vi "多参数测量数据存储.vi"(5 "数据类型":string(combo)="N", 6 "手动启动标记":bool, 7 "测量模式":T2(ring)=enum."水样测试", 8 "error in (no error)":errorcluster, 9 "database":string, 10 "table输入":string, 11 "data in":T1) -> (0 "error out":errorcluster)   [LabVIEW 2016, in "斯坦道多参数.lvlib"]
uses:
  <vilib>/Utility/sysdir.llb/System Directory Type.ctl
  <vilib>/Utility/error.llb/DialogType.ctl
  <vilib>/addons/database/Auxilliary.llb/DB Tools Transaction.ctl
  <vilib>/addons/database/Auxilliary.llb/DB Tools Isolation Level.ctl
  <vilib>/addons/database/Connection.llb/DB Tools Open Connec (String).vi
  <vilib>/addons/database/Connection.llb/Conn Execute.vi
  <vilib>/addons/database/Recordset.llb/Rec Destroy - Connection.vi
  <vilib>/addons/database/Connection.llb/Conn Transaction.vi
  <vilib>/addons/database/NI_Database_API.lvlib
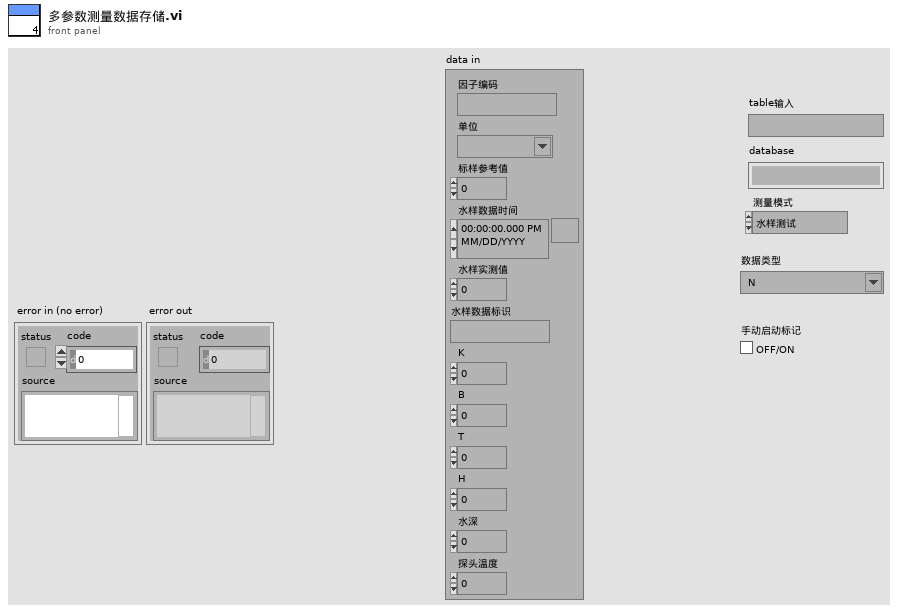
[diagram p1: front panel]
types:
  T1 = cluster{"因子编码":string, "单位":string, "标样参考值":sgl, "水样数据时间":timestamp, "水样实测值":sgl, "水样数据标识":string, "K":sgl, "B":sgl, "T":sgl, "H":sgl, "水深":sgl, "探头温度":sgl}
  T2 = enum16{"待机", "水样测试", "标样核查", "零点核查", "跨度核查", "空白测试", "平行样测试", "加标回收", "空白校准", "标样校准", "初始化（清洗）"}
  T3 = typedef "NI_Database_API.lvlib/DB Tools Transaction.ctl" = enum16{"begin", "commit", "rollback"}
  T4 = typedef "NI_Database_API.lvlib/DB Tools Isolation Level.ctl" = enum16{"chaos", "read uncommitted", "read committed", "repeatable read", "serializable"}
  T5 = typedef "DialogType.ctl" = u16
  T6 = typedef "System Directory Type.ctl" = i32
  T7 = cluster{"时间标识":timestamp, "测量模式":string, "数据类型":string, "监测值":sgl, "单位":string, "数据标识":string, "因子编码":string, "标样参考值":sgl, "K":sgl, "B":sgl, "温度":sgl, "湿度":sgl, "水深":sgl, "探头温度":sgl, "LastTime":timestamp}
  T8 = typedef "NI_Database_API.lvlib/Conn ObjectReference.ctl" = refnum<k1>
  T9 = typedef "NI_Database_API.lvlib/Rec ObjectReference.ctl" = refnum<k1>
  T10 = cluster{"时间标识":timestamp, "设备":string, "日志信息":string}
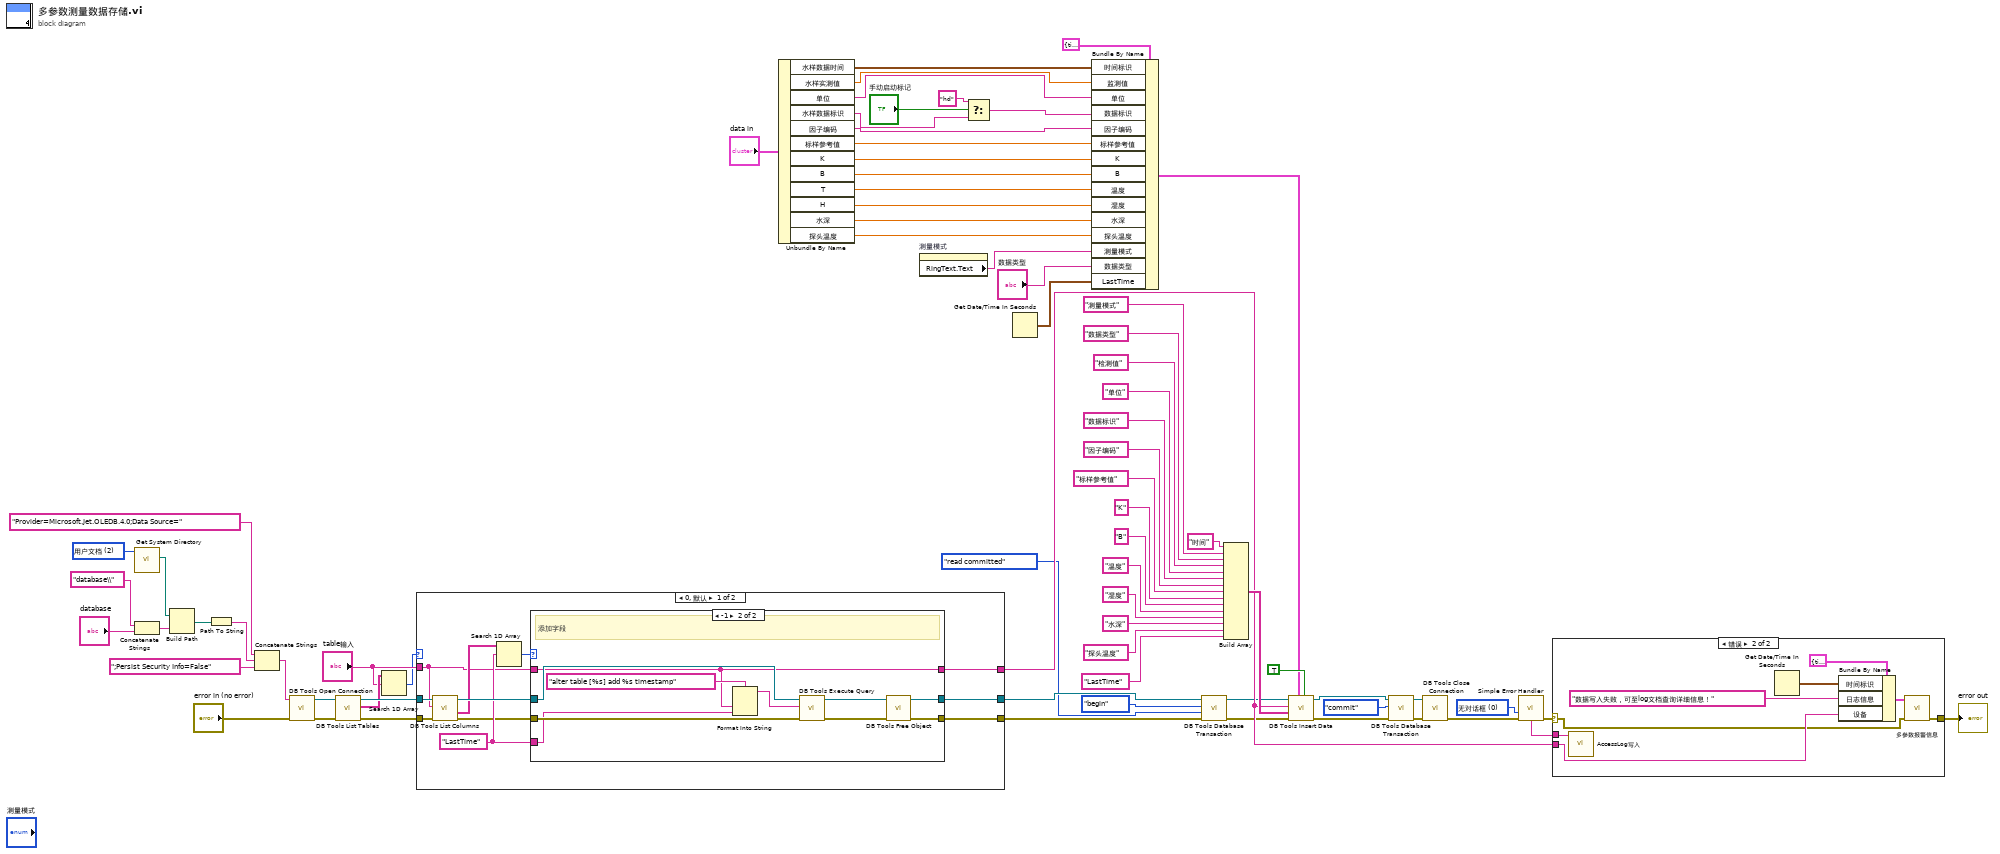
[diagram p0: block diagram]
diagram:
  w27 = T5 0 items=["无对话框", "确定信息", "继续或停止信息", "确定信息＋警告", "继续/停止+警告"] ("type of dialog (OK msg:1)")
  w47 = T6 2 items=["用户目录"=0, "用户桌面"=1, "用户文档"=2, "用户应用程序数据"=3, "用户设置"=4, "用户临时目录"=5, "公共文档"=6, "公共应用程序数据"=7, "公共设置"=8, "公共缓存"=13, "系统核心库"=9, "系统安装库"=10, "应用程序文件"=11, "启动盘根目录"=12] ("system directory type")
  n1 = call <vilib>:"Get System Directory.vi"("system directory type"=w47) -> ("system directory"=w45:path)  [unwired: 10 in]
  n2 = Concatenate Strings("database\\" ("condition"), "database") -> (w39:string)
  n3 = Build Path(base path=w45, name or relative path=w39) -> (appended path=w44:path)
  n4 = Path To String(path=w44) -> (string=w43:string)
  n5 = Concatenate Strings("Provider=Microsoft.Jet.OLEDB.4.0;Data Source=" ("condition"), w43, ";Persist Security Info=False" ("condition")) -> (w41:string)
  n6 = call-poly <vilib>:"DB Tools Open Connection.vi"("error in (no error)"="error in (no error)", "connection information"=w41) -> ("error out"=w18:errorcluster, "connection reference"=w29:T8)  [unwired: 6 in]
  n7 = call <vilib>:"DB Tools List Tables.vi"("error in (no error)"=w18, "connection reference"=w29) -> ("error out"=w17:errorcluster, "tables"=w16:string[], "connection reference out"=w19:T8)  [unwired: 3 in]
  n8 = Search 1D Array(1D array=w16, element="table输入") -> (index of element=w14:i32)  [unwired: 1 in]
  n9 = case shown="0, 默认" w14 {
    tunnel: [w79 w100] -> w28
    tunnel: [w78 w98] -> w10
    tunnel: [w77 w99] -> w22
    tunnel: w19 -> [w76 w100]
    tunnel: w17 -> [w75 w98]
    tunnel: "table输入" -> [w74 w99]
    frame 0, Default {
      w83 = "LastTime" ("元素")
      n10 = call <vilib>:"DB Tools List Columns.vi"("error in (no error)"=w75, "table"=w74, "connection reference"=w76) -> ("error out"=w81:errorcluster, "columns"=w82:string[], "connection reference out"=w84:T8)  [unwired: 1 in, 1 out]
      n11 = Search 1D Array(1D array=w82, element=w83) -> (index of element=w80:i32)  [unwired: 1 in]
      n12 = case shown="-1" w80 {
        tunnel: w84 -> [w87 w95]
        tunnel: w81 -> [w86 w94]
        tunnel: w83 -> [_ w92]
        tunnel: [w87 w90] -> w79
        tunnel: [w86 w89] -> w78
        tunnel: w74 -> [w85 w88]
        tunnel: [w85 w88] -> w77
        frame 0, Default {
        }
        frame -1 {
          # "添加字段"
          n13 = Format Into String(format string="alter table [%s] add %s timestamp", w88, w92) -> (resulting string=w91:string)  [unwired: 2 in, 1 out]
          n14 = call-poly <vilib>:"DB Tools Execute Query.vi"("error in (no error)"=w94, "SQL query"=w91, "connection reference"=w95) -> ("error out"=w96:errorcluster, "recordset reference"=w97:T9)  [unwired: 5 in]
          n15 = call-poly <vilib>:"DB Tools Free Object.vi"("error in (no error)"=w96, "recordset reference"=w97) -> ("error out"=w89:errorcluster, "connection reference"=w90:T8)  [unwired: 8 in]
        }
      }
    }
    frame -1 {
    }
  }
  n16 = Unbundle By Name("data in") -> ("水样数据时间"=w64:timestamp, "水样实测值"=w63:sgl, "单位"=w56:string, "水样数据标识"=w1:string, "因子编码"=w55:string, "标样参考值"=w57:sgl, "K"=w58:sgl, "B"=w62:sgl, "T"=w61:sgl, "H"=w60:sgl, "水深"=w35:sgl, "探头温度"=w32:sgl)
  n17 = property on="测量模式" class="Enum (严格)"() -> ("RingText.Text"=w54:string)  [unwired: 2 in, 2 out]
  n18 = Select(t="hd", s="手动启动标记", f=w1) -> (s? t:f=w3:string)
  n19 = Get Date/Time In Seconds() -> (seconds since 1Jan1904=w21:timestamp)
  n20 = Bundle By Name(cluster=T7 {"时间标识"=timestamp(0 s since 1904-01-01), "测量模式"="", "数据类型"="", "监测值"=0.0, "单位"="", "数据标识"="", "因子编码"="", "标样参考值"=0.0, "K"=0.0, "B"=0.0, "温度"=0.0, "湿度"=0.0, "水深"=0.0, "探头温度"=0.0, "LastTime"=timestamp(0 s since 1904-01-01)} ("data输出"), "时间标识"=w64, "监测值"=w63, "单位"=w56, "数据标识"=w3, "因子编码"=w55, "标样参考值"=w57, "K"=w58, "B"=w62, "温度"=w61, "湿度"=w60, "水深"=w35, "探头温度"=w32, "测量模式"=w54, "数据类型"="数据类型", "LastTime"=w21) -> (w36:T7)
  n21 = call-poly <vilib>:"DB Tools Database Transaction.vi"("error in (no error)"=w10, "isolation level (chaos)"=DB_Tools_Isolation_Level."read committed", "operation (begin)"=DB_Tools_Transaction."begin", "connection reference"=w28) -> ("error out"=w9:errorcluster, "connection reference out"=w13:T8)  [unwired: 2 in]
  n22 = Build Array("时间", "测量模式", "数据类型", "检测值", "单位", "数据标识", "因子编码", "标样参考值", "K", "B", "温度", "湿度", "水深", "探头温度", "LastTime") -> (w37:string[])
  n23 = call <vilib>:"DB Tools Insert Data.vi"("create table? (F)"=TRUE, "data"=w36, "error in (no error)"=w9, "columns"=w37, "table"=w22, "connection reference"=w13) -> ("error out"=w7:errorcluster, "connection reference out"=w49:T8)  [unwired: 4 in]
  n24 = call-poly <vilib>:"DB Tools Database Transaction.vi"("error in (no error)"=w7, "operation (begin)"=DB_Tools_Transaction."commit", "connection reference"=w49) -> ("error out"=w6:errorcluster, "connection reference out"=w8:T8)  [unwired: 3 in]
  n25 = call <vilib>:"DB Tools Close Connection.vi"("error in (no error)"=w6, "connection reference"=w8) -> ("error out"=w24:errorcluster)  [unwired: 5 in]
  n26 = call <vilib>:"Simple Error Handler.vi"("type of dialog (OK msg:1)"=w27, "error in (no error)"=w24) -> ("error out"=w25:errorcluster, "message"=w26:string)  [unwired: 3 in, 3 out]
  n27 = case shown="错误" w25 {
    selector: w25 -> [w101 w102]
    tunnel: w26 -> [_ w104]
    tunnel: [w101 w107] -> w23
    tunnel: w22 -> [_ w106]
    frame No Error {
    }
    frame Error {
      n28 = call "AccessLog写入.vi"("Log"=w104) -> ()  [unwired: 11 in]
      n29 = Get Date/Time In Seconds() -> (seconds since 1Jan1904=w105:timestamp)
      n30 = Bundle By Name(cluster=T10 {"时间标识"=timestamp(0 s since 1904-01-01), "设备"="", "日志信息"=""} ("data in"), "时间标识"=w105, "日志信息"="数据写入失败，可至log文档查询详细信息！", "设备"=w106) -> (w108:T10)
      n31 = call "多参数报警信息.vi"("error in (no error)"=w102, "data in"=w108) -> ("error out"=w107:errorcluster)  [unwired: 9 in]
    }
  }
  "error out" <- w23
